vi "Get configuration chain.vi"(8 "error in (no error)":errorcluster, 11 "Cascade512Base in":refnum<class "DAQCascade512.lvclass">) -> (0 "error out":errorcluster, 1 "class name":string[](array[string]), 2 "configuration chain":variant[](array[variant]), 3 "Cascade512Base out":refnum<class "DAQCascade512.lvclass">)   [LabVIEW 2012, in "DAQCascade512.lvclass"]
doc: "Returns an array of variants containing the configuration clusters of each class in the inheritance chain (lowest child class first), together with an array of all class names in the inheritance chain.\n\nFor classes without configuration cluster, the configuration chain contains empty variants."
uses:
  DAQCascade512.lvclass
  <vilib>/Distrio/Murmex/Murmex/Murmex.lvclass
  DAQCascade512.lvclass/DAQCascade512.ctl
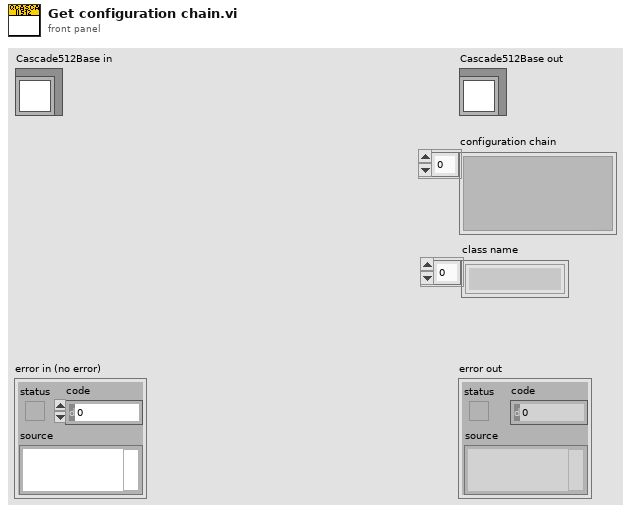
[diagram p1: front panel]
types:
  T1 = typedef "Clearing_mode.ctl" = dbl
  T2 = typedef "Readout_mode.ctl" = dbl
  T3 = typedef "ADC_gain.ctl" = i32
  T4 = typedef "Image_type.ctl" = u32
  T5 = cluster{"Camera configuration":cluster{"Temperature":dbl, "EMGain":dbl, "ClearMode":T1, "ReadoutMode":T2, "ADC Gain":T3}, "Acqusition Info":cluster{"Image type":T4, "Acquire / Focus Flag":u32}}
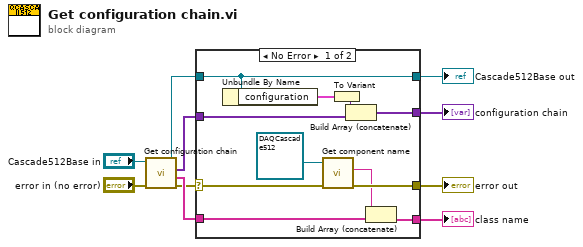
[diagram p0: block diagram]
diagram:
  n1 = call-parent "Get configuration chain.vi"("error in (no error)"="error in (no error)", "MurmexBase in"="Cascade512Base in") -> ("error out"=w2:errorcluster, "class name"=w4:string[], "configuration chain"=w6:variant[], "MurmexBase out"=w8:refnum<class "DAQCascade512.lvclass">)  [unwired: 6 in]
  n2 = case shown="No Error" w2 {
    selector: w2 -> [w17 w24]
    tunnel: w8 -> [w13 w23]
    tunnel: [w13 w23] -> w7
    tunnel: w6 -> [w21 w22]
    tunnel: [w20 w22] -> w1
    tunnel: [w18 w24] -> w5
    tunnel: w4 -> [w16 w25]
    tunnel: [w15 w25] -> w3
    frame No Error {
      n3 = Unbundle By Name(w13) -> ("configuration"=w12:T5)
      n4 = call <vilib>:"Get component name.vi"("error in (no error)"=w17, "Murmex in"=refnum<class "DAQCascade512.lvclass"> refnum ("DAQCascade512")) -> ("error out"=w18:errorcluster, "component name"=w14:string)  [unwired: 7 in, 1 out]
      n5 = To Variant(anything=w12) -> (Variant=w11:variant)
      n6 = Build Array (concatenate)(w11, w21) -> (w20:variant[])
      n7 = Build Array (concatenate)(w14, w16) -> (w15:string[])
    }
    frame Error {
    }
  }
  "error out" <- w5
  "Cascade512Base out" <- w7
  "configuration chain" <- w1
  "class name" <- w3
